vi "Get Result.vi"(8 "error in (no error)":errorcluster, 11 "LakeShore370 in":refnum<class "LakeShore370.lvclass">) -> (0 "error out":errorcluster, 2 "Mag Lab Result.lvclass":refnum<class "Mag Lab Result.lvclass">, 3 "LakeShore370 out":refnum<class "LakeShore370.lvclass">)   [LabVIEW 2015, in "LakeShore370.lvclass"]
uses:
  LakeShore370.lvclass
  Mag Lab Result/Mag Lab Result.lvclass
  Mag Lab Hardware.lvclass/Mag Lab Hardware.ctl
  Mag Lab Root/Mag Lab Root.lvclass/Mag Lab Root.ctl
  Instruments/LakeShore/LakeShore370/Get LakeShore 370 Resistance_VISA.vi
  Mag Lab Hardware.lvclass
  Mag Lab Error Handler/Mag Lab Error Handler.lvclass
  Mag Lab Root/Mag Lab Root.lvclass
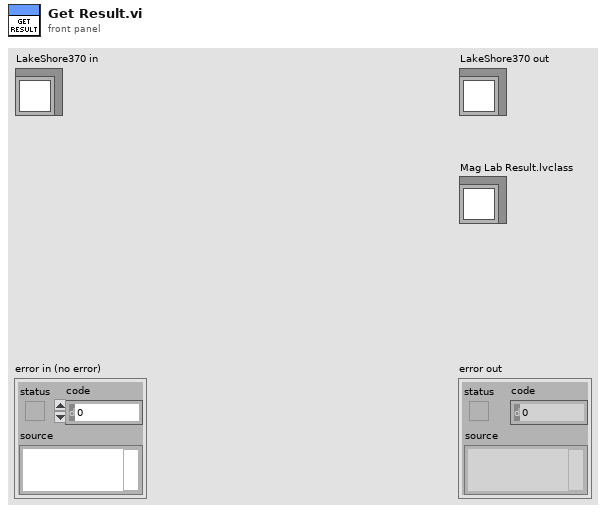
[diagram p1: front panel]
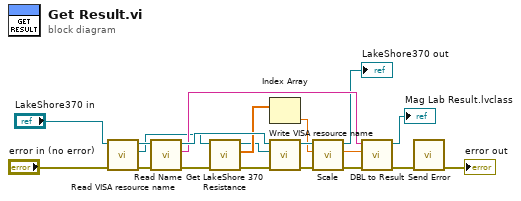
[diagram p0: block diagram]
diagram:
  n1 = call "Read VISA resource name.vi"("error in (no error)"="error in (no error)", "Mag Lab Hardware in"="LakeShore370 in") -> ("error out"=w19:errorcluster, "VISA resource name"=w6:refnum<visa-resource-name>, "Mag Lab Hardware out"=w20:refnum<class "LakeShore370.lvclass">)  [unwired: 7 in]
  n2 = call "Read Name.vi"("error in (no error)"=w19, "Mag Lab Root in"=w20) -> ("error out"=w3:errorcluster, "Name"=w16:string, "Mag Lab Root out"=w18:refnum<class "LakeShore370.lvclass">)  [unwired: 7 in]
  n3 = call-poly "Get LakeShore 370 Resistance.vi"("error in (no error)"=w3, "VISA resource name"=w6) -> ("error out"=w2:errorcluster, "Resistance"=w5:dbl[], "VISA resource name out"=w1:refnum<visa-resource-name>)  [unwired: 7 in]
  n4 = Index Array(array=w5) -> (element=w4:dbl)  [unwired: 1 in]
  n5 = call "Write VISA resource name.vi"("error in (no error)"=w2, "VISA resource name"=w1, "Mag Lab Hardware in"=w18) -> ("error out"=w12:errorcluster, "Mag Lab Hardware out"=w17:refnum<class "LakeShore370.lvclass">)  [unwired: 7 in]
  n6 = call-dynamic "Scale.vi"("error in (no error)"=w12, "Input"=w4, "Meter in"=w17) -> ("error out"=w13:errorcluster, "Output"=w14:dbl, "Meter out"=→"LakeShore370 out":refnum<class "LakeShore370.lvclass">)  [unwired: 6 in]
  n7 = call "DBL to Result.vi"("error in (no error)"=w13, "Data"=w14, "Name"=w16) -> ("error out"=w15:errorcluster, "Mag Lab Result out"=→"Mag Lab Result.lvclass":refnum<class "Mag Lab Result.lvclass">)  [unwired: 7 in]
  n8 = call "Send Error.vi"("error in (no error)"=w15) -> ("error out"=→"error out":errorcluster)  [unwired: 9 in, 1 out]
